vi "Mixer.Set Channel Property.vi"(0 "channel":string, 5 "property":string, 7 "value":bool) -> ()   [LabVIEW 2020]
uses:
  Typedefs/Mixer.Channel Property Data.ctl
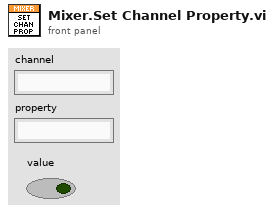
[diagram p1: front panel]
types:
  T1 = typedef "Mixer.Channel Property Data.ctl" = cluster{"channel":string, "property":string, "value":bool}
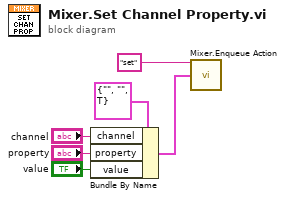
[diagram p0: block diagram]
diagram:
  n1 = Bundle By Name(cluster=T1 {"channel"="", "property"="", "value"=TRUE} ("Cluster"), "channel"="channel", "property"="property", "value"="value") -> (w1:T1)
  n2 = call "Mixer.Enqueue Action.vi"("action"="set", "data"=w1) -> ()  [unwired: 13 in, 1 out]
